vi "VALEW_ATC_Calc Inlet Temps.vi"(5 "T(warm measured)":dbl, 7 "T(cold measured)":dbl, 9 "T(hot measured)":dbl) -> (6 "T(cold calculated)":dbl, 10 "T(hot calculated)":dbl)   [LabVIEW 2016, in "2015 VA Washer.lvlib"]
uses:
  Projects/2015 VA Washer.lvlib
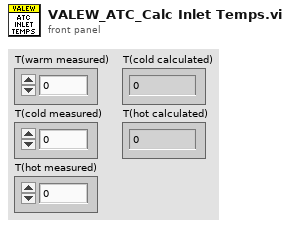
[diagram p1: front panel]
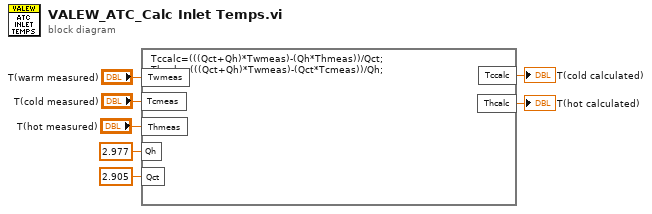
[diagram p0: block diagram]
diagram:
  n1 = formula code="Tccalc=(((Qct+Qh)*Twmeas)-(Qh*Thmeas))/Qct;\nThcalc=(((Qct+Qh)*Twmeas)-(Qct*Tcmeas))/Qh;"("Twmeas"="T(warm measured)", "Tcmeas"="T(cold measured)", "Qh"=2.977 ("input variable"), "Qct"=2.905 ("input variable"), "Thmeas"="T(hot measured)") -> ("Tccalc"=→"T(cold calculated)":dbl, "Thcalc"=→"T(hot calculated)":dbl)
